vi "QR decomposition update by Givens rotation.vi"() -> ()   [LabVIEW 2023]
doc: "This example generates a random <b>n</b>-by-<b>n</b> matrix as the <b>Input Matrix</b> and performs a QR decomposition of <b>Input Matrix</b> by either Givens rotation or fast Givens rotation. Matrix <b>R</b> is the resulting upper triangular matrix."
uses:
  <vilib>/Analysis/BLAS.llb/drotg - Givens Rotation Parameters (DBL).vi
  <vilib>/Analysis/BLAS.llb/drot - Givens Rotation (DBL).vi
  <vilib>/Analysis/NI_AALBLAS.lvlib
  <vilib>/Analysis/NI_AALBase.lvlib
panel:
  in  "Tab Control":T1(tab)
  in  "n":i32=6
  in  "method":u16(ring) items=["Givens", "Fast Givens"]
  out "R":dbl[][](array[numeric]) format="%#.6f"
  out "Input Matrix":dbl[][](array[numeric]) format="%#.6f"
  # "Overview: Demonstrates the use of the Basic Linear Algebra Subroutines (BLAS) VIs to compute the QR decomposition of a matrix.\nRequirements: LabVIEW Full Development System\nInstructions: \n1. Run the VI.\n2. Observe the resulting R matrix.\n3. Change the values of n and method and run the VI again. Observe the new results in the R matrix."
  # "1) Calculate the Givens rotation parameters c and s  by the X[N-1,j] and X[N-2,j], j starts from 0.\n2) Zero X[N-1,j] by the resulting Givens rotation parameters.\n3) Repeat step 1,2 (N-1-j) times, and zero the  (N-1-j) nether elements in this column.\n4) Increase j by 1, and repeat step 1, 2, 3 to zero the nether elements in the next column.\n5) When j is equal to N-2, the resulting matrix is an upper triangular matrix."
  # "1) Calculate the fast Givens rotation matrix H by X[N-1,j] and X[N-2,j], j starts from 0.\n2) Zero X[N-1,j] by the resulting fast Givens rotation matrix.\n3) Repeat step 1 and step 2 (N-1-j) times, and zero the  (N-1-j) nether elements in this column.\n4) Increase j by 1, and repeat step 1, 2, 3 to zero the nether elements in the next column.\n5) When j is equal to N-2, the matrix is an upper triangular matrix."
  # "and"
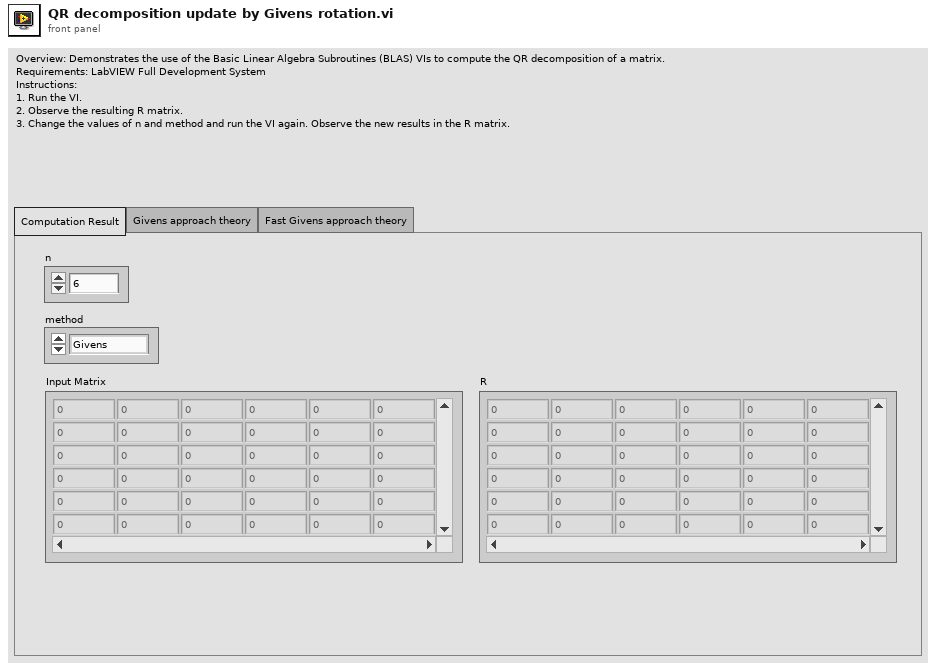
[diagram p1: front panel]
types:
  T1 = enum32{"Computation Result", "Givens approach theory", "Fast Givens approach theory"}
  T2 = typedef "NI_Matrix.lvlib/RealMatrix.ctl" = dbl[][]
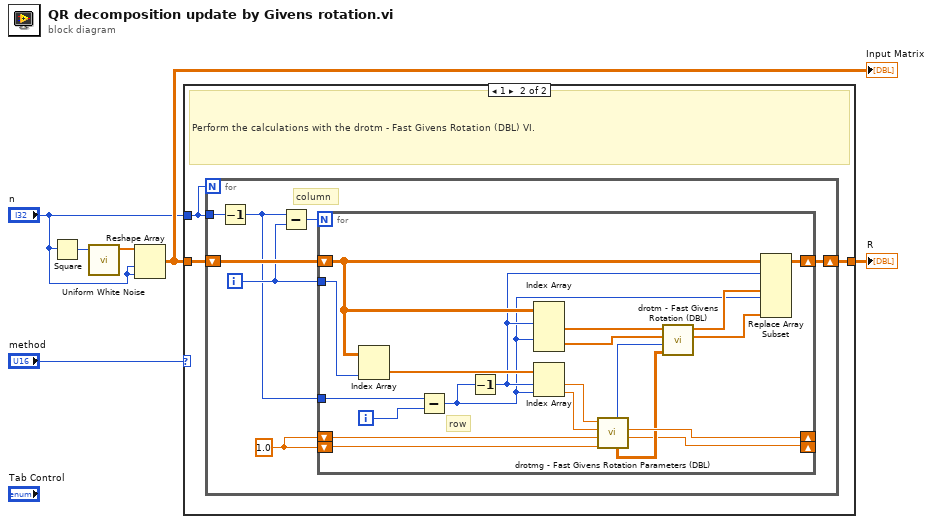
[diagram p0: block diagram]
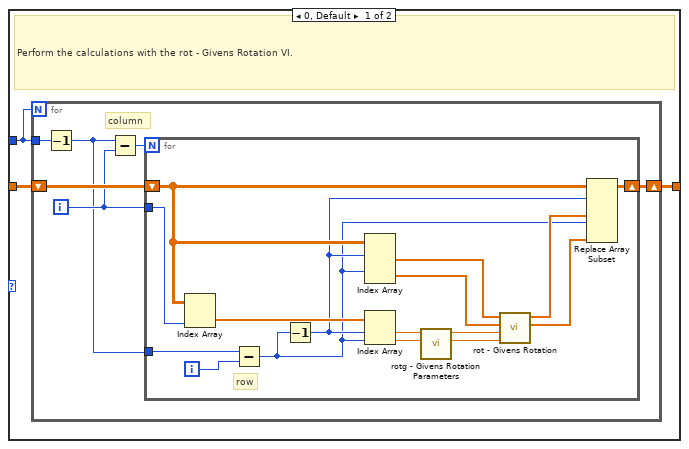
[diagram p2: hidden frame]
diagram:
  n1 = Square(x="n") -> (x^2=w6:i32)
  n2 = call <vilib>:"Uniform White Noise.vi"("samples"=w6) -> ("uniform white noise"=w5:dbl[])  [unwired: 9 in, 1 out]
  n3 = Reshape Array(w5, "n", "n") -> (w3:dbl[][])
  "Input Matrix" <- w3
  n4 = case shown="1" "method" {
    tunnel: "n" -> [w7 w32]
    tunnel: w3 -> [w8 w34]
    tunnel: [w9 w33] -> w2
    frame 0, Default {
      # "Perform the calculations with the rot - Givens Rotation VI."
      n5 = for {
        N: w7 -> [_]
        tunnel: w7 -> [w15]
        shift-right: [w14] -> w9
        shift-left: w8 -> [w13]
        i -> [w11]
        # "column"
        n6 = Decrement(x=w15) -> (x-1=w10:i32)
        n7 = Subtract(x=w10, y=w11) -> (x-y=w12:i32)
        n8 = for {
          N: w12 -> [_]
          shift-right: [w20] -> w14
          shift-left: w13 -> [w27]
          tunnel: w11 -> [w30]
          tunnel: w10 -> [w23]
          i -> [w28]
          # "row"
          n9 = Index Array(array=w27, index (col)=w30) -> (element=w29:dbl[])  [unwired: 1 in]
          n10 = Subtract(x=w23, y=w28) -> (x-y=w21:i32)
          n11 = Decrement(x=w21) -> (x-1=w24:i32)
          n12 = Index Array(array=w27, index (row) #1=w24, index (row) #2=w21) -> (element #1=w26:dbl[], element #2=w25:dbl[])  [unwired: 2 in]
          n13 = Index Array(array=w29, index #1=w24, index #2=w21) -> (element #1=w19:dbl, element #2=w18:dbl)
          n14 = call-poly <vilib>:"rotg - Givens Rotation Parameters.vi"("y"=w18, "x"=w19) -> ("s"=w16:dbl, "c"=w17:dbl)  [unwired: 8 out]
          n15 = call-poly <vilib>:"rot - Givens Rotation.vi"("s"=w16, "c"=w17, "y in"=w25, "x in"=w26) -> ("y out"=w22:dbl[], "x out"=w31:dbl[])  [unwired: 2 in, 4 out]
          n16 = Replace Array Subset(array=w27, new element #1=w31, index (row) #1=w24, new element #2=w22, index (row) #2=w21) -> (w20:dbl[][])  [unwired: 2 in]
        }
      }
    }
    frame 1 {
      # "Perform the calculations with the drotm - Fast Givens Rotation (DBL) VI."
      n17 = for {
        N: w32 -> [_]
        tunnel: w32 -> [w41]
        shift-right: [w40] -> w33
        shift-left: w34 -> [w39]
        i -> [w37]
        w35 = 1.0
        # "column"
        n18 = Decrement(x=w41) -> (x-1=w36:i32)
        n19 = Subtract(x=w36, y=w37) -> (x-y=w38:i32)
        n20 = for {
          N: w38 -> [_]
          shift-right: [w45] -> w40
          shift-left: w39 -> [w55]
          tunnel: w37 -> [w60]
          tunnel: w36 -> [w51]
          shift-right: [w49] -> _
          shift-left: w35 -> [w50]
          shift-right: [w43] -> _
          shift-left: w35 -> [w42]
          i -> [w58]
          # "row"
          n21 = Index Array(array=w55, index (col)=w60) -> (element=w59:dbl[])  [unwired: 1 in]
          n22 = Subtract(x=w51, y=w58) -> (x-y=w47:i32)
          n23 = Decrement(x=w47) -> (x-1=w52:i32)
          n24 = Index Array(array=w55, index (row) #1=w52, index (row) #2=w47) -> (element #1=w54:dbl[], element #2=w53:dbl[])  [unwired: 2 in]
          n25 = Index Array(array=w59, index #1=w52, index #2=w47) -> (element #1=w57:dbl, element #2=w56:dbl)
          n26 = call <vilib>:"drotmg - Fast Givens Rotation Parameters (DBL).vi"("d2 in"=w42, "d1 in"=w50, "y"=w56, "x"=w57) -> ("d2 out"=w43:dbl, "d1 out"=w49:dbl, "Rotation Matrix"=w48:T2, "rotation matrix flag"=w44:i32)  [unwired: 4 out]
          n27 = call <vilib>:"drotm - Fast Givens Rotation (DBL).vi"("Rotation Matrix"=w48, "rotation matrix flag"=w44, "y in"=w53, "x in"=w54) -> ("y out"=w46:dbl[], "x out"=w61:dbl[])  [unwired: 2 in, 4 out]
          n28 = Replace Array Subset(array=w55, new element #1=w61, index (row) #1=w52, new element #2=w46, index (row) #2=w47) -> (w45:dbl[][])  [unwired: 2 in]
        }
      }
    }
  }
  "R" <- w2
